vi "ProdaNG.FreeStructArray.vi"(8 "error in (no error)":errorcluster, 10 "Pointers":u32[](array[numeric])) -> (0 "error out":errorcluster)   [LabVIEW 2016]
doc: "This function releases the memory of Arrays, which is allocated by the DLL. \nParameter:\narrayOfPtrs is an Array pointer that has been filled by DLL functions, which pass back result lists. After calling this function, the content of this parameter is invalid and must not be used any further on."
uses:
  prodllNG.dll
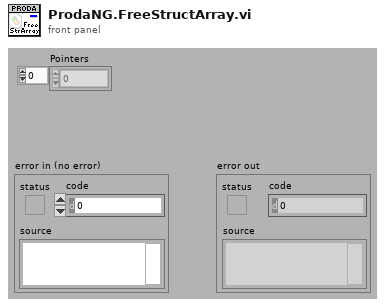
[diagram p1: front panel]
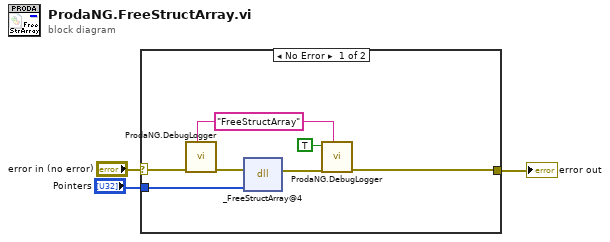
[diagram p0: block diagram]
diagram:
  n1 = case shown="No Error" "error in (no error)" {
    selector: "error in (no error)" -> [w4 w11]
    tunnel: [w6 w11] -> w2
    tunnel: "Pointers" -> [w10 _]
    frame No Error {
      w9 = "FreeStructArray" ("cmd")
      n2 = call "ProdaNG.DebugLogger.vi"("cmd"=w9, "error in (no error)"=w4) -> ("error out"=w5:errorcluster)  [unwired: 9 in]
      n3 = dll-call lib="D:/Maszup/WABCO/SVN/LineTraceSystem/SOFTWARE/sources/Database/ProdaNG/prodllNG.dll" fn="_FreeStructArray@4" ("ProDll.dll:InitProDll")(error in=w5, "arrayOfPtrs"=w10) -> (error out=w7:errorcluster)  [unwired: 4 in, 1 out]
      n4 = call "ProdaNG.DebugLogger.vi"("cmd"=w9, "error in (no error)"=w7, "done? (F)"=TRUE) -> ("error out"=w6:errorcluster)  [unwired: 8 in]
    }
    frame Error {
    }
  }
  "error out" <- w2
